vi "colors.vi"(1 "colors needed":i16) -> (0 "colors":u32[](array[colorbox])=[16717824, 16775680, 65289, 1442031, 16711898, 9306367, 16711704, 16773418, 4914944, 65469, 18175, 15805183, 16711776, 16745216, 16773632, 7396352, 62719, 16383, 15925503, 16711686, 16775954, 65372, 51354, 19711, 7082751, 15663288, 16711680, 11468586, 52719, 1214975, 16711830])   [LabVIEW 2012]
panel:
  out "total":i32
  out "number":i32
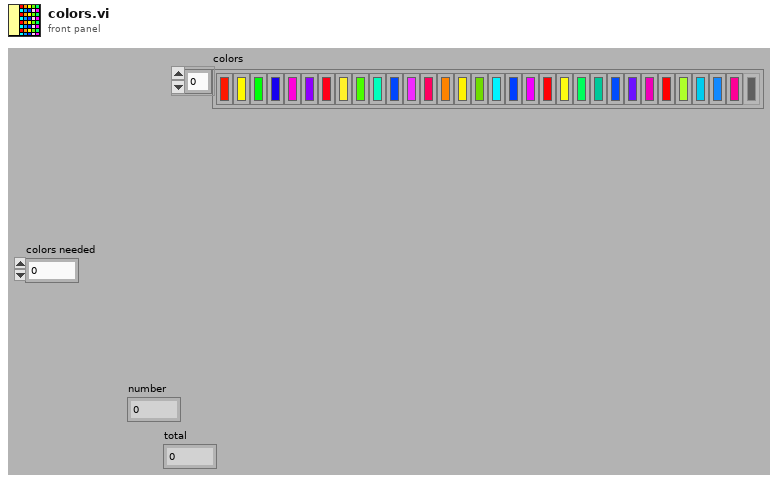
[diagram p1: front panel]
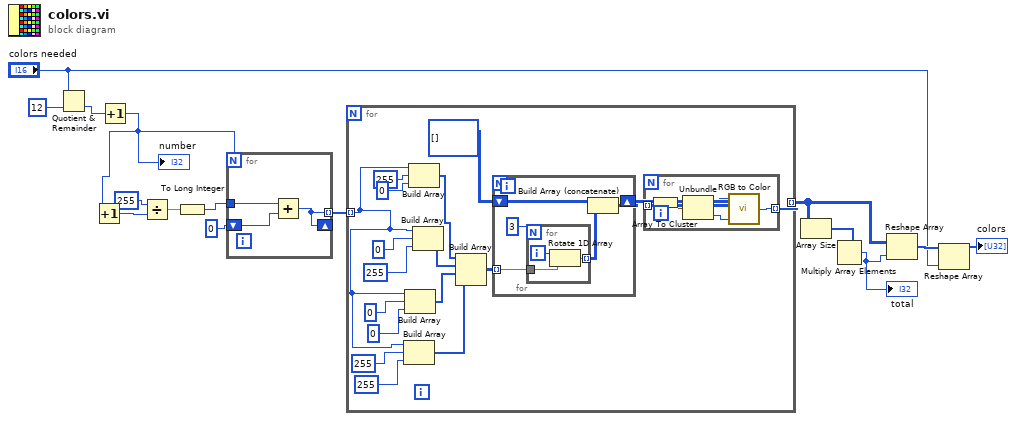
[diagram p0: block diagram]
diagram:
  n1 = Quotient & Remainder(x="colors needed", y=i16 12) -> (floor(x/y)=w5:i16)  [unwired: 1 out]
  n2 = Increment(x=w5) -> (x+1=w4:i16)
  "number" <- w4
  n3 = Increment(x=w4) -> (x+1=w12:i16)
  n4 = Divide(x=255, y=w12) -> (x/y=w14:dbl)
  n5 = To Long Integer(number=w14) -> (32bit integer=w13:i32)
  n6 = for {
    N: w4 -> [_]
    shift-right: [w17] -> _
    shift-left: 0 -> [w18]
    tunnel: [w17] -> w10 mode=indexing
    tunnel: w13 -> [w16]
    n7 = Add(x=w16, y=w18) -> (x+y=w17:i32)
  }
  n8 = for {
    tunnel: w10 -> [w25] mode=indexing
    tunnel: [w35] -> w8 mode=indexing
    n9 = Build Array(w25, 255, 255) -> (w27:i32[])
    n10 = Build Array(w25, 0, 0) -> (w28:i32[])
    n11 = Build Array(w25, 255, 0) -> (w22:i32[])
    n12 = Build Array(w25, 0, 255) -> (w26:i32[])
    n13 = Build Array(w22, w26, w28, w27) -> (w21:i32[][])
    n14 = for {
      tunnel: w21 -> [w40] mode=indexing
      shift-right: [w37] -> w19
      shift-left: i32[][] [] -> [w36]
      n15 = for {
        N: 3 -> [_]
        tunnel: [w43] -> w38 mode=indexing
        tunnel: w40 -> [w42]
        i -> [w41]
        n16 = Rotate 1D Array(1:w42, 2:w41) -> (0:w43:i32[])
      }
      n17 = Build Array (concatenate)(w36, w38) -> (w37:i32[][])
    }
    n18 = for {
      tunnel: [w45] -> w35 mode=indexing
      tunnel: w19 -> [w46] mode=indexing
      n19 = Array To Cluster(array=w46) -> (cluster=w49:cluster{"[0]":i32, "[1]":i32, "[2]":i32})
      n20 = Unbundle(w49) -> ("[0]"=w48:i32, "[1]"=w47:i32, "[2]"=w44:i32)
      n21 = call <vilib>:"RGB to Color.vi"("B"=w44, "G"=w47, "R"=w48) -> ("Color"=w45:u32)
    }
  }
  n22 = Array Size(array=w8) -> (size(s)=w9:i32[])
  n23 = Multiply Array Elements(1:w9) -> (0:w7:i32)
  "total" <- w7
  n24 = Reshape Array(w8, w7) -> (w3:u32[])
  n25 = Reshape Array(w3, "colors needed") -> (→"colors":u32[])
